vi "Edit Options.vi"(8 "error in (no error)":errorcluster, 11 "Config":T1) -> (0 "error out":errorcluster, 2 "OK?":bool, 3 "Config out":T1)   [LabVIEW 2023, in "VI Properties Editor.lvlib"]
doc: "Displays a window to edit various options present in the tool."
uses:
  VI Properties Editor.lvlib
  CTLs/Config.ctl
panel:
  in  "Abbreviate Names?":bool caption="Abbreviate names"
  in  "Format Bold Tags?":bool caption="Format bold text tags"
  in  "Show Conpane Ctls Only?":bool caption="Show connector pane controls only"
  in  "Confirm Revert All?":bool caption="Confirm Revert All action"
  in  "Confirm Revert?":bool caption="Confirm Revert action"
  in  "Confirm Save All?":bool caption="Confirm Save All action"
  in  "Confirm Save?":bool caption="Confirm Save action"
  in  "Cancel":bool
  in  "OK":bool
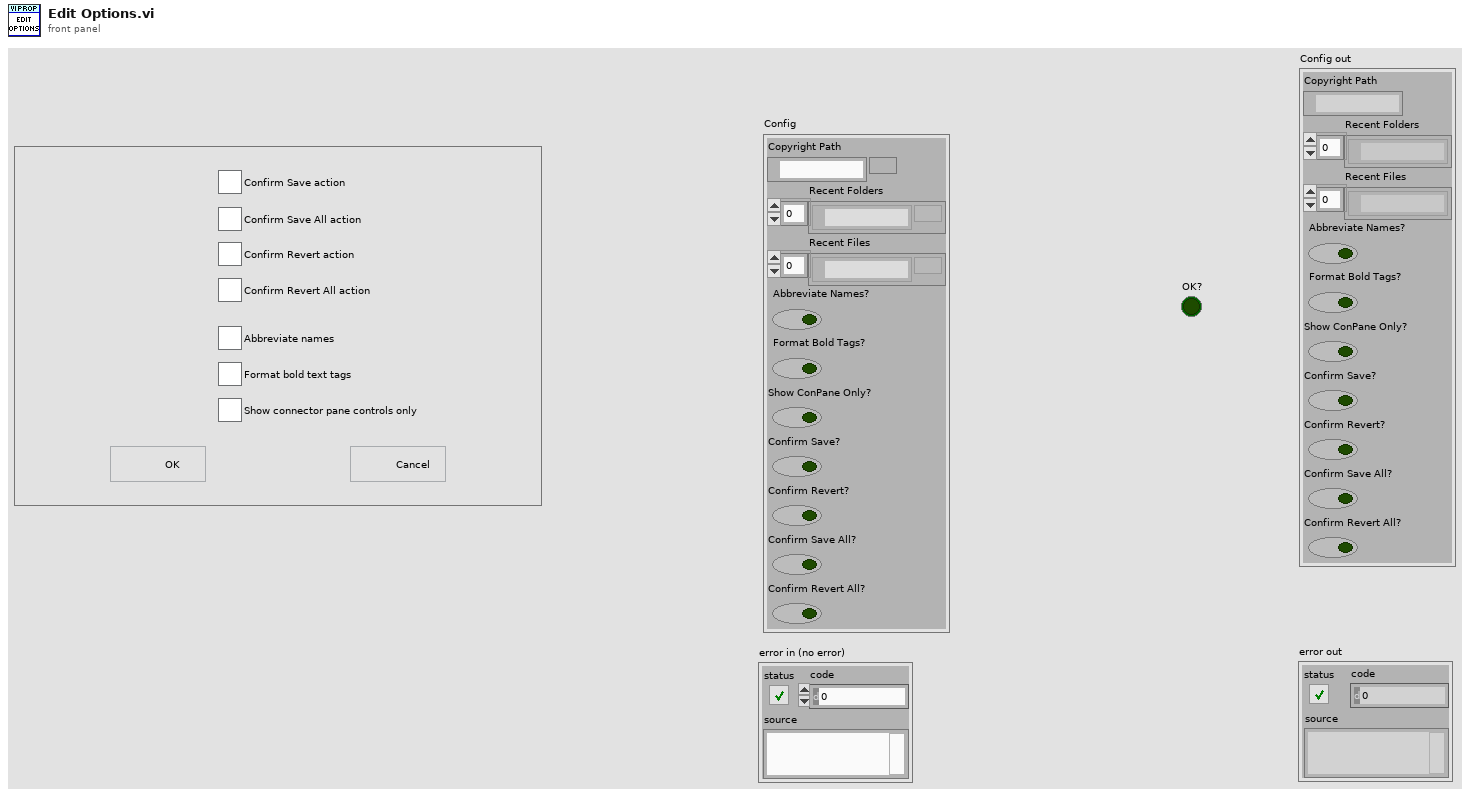
[diagram p1: front panel]
types:
  T1 = typedef "VI Properties Editor.lvlib/Config.ctl" = cluster{"Copyright Path":path, "Recent Folders":path[], "Recent Files":path[], "Abbreviate Names?":bool, "Format Bold Tags?":bool, "Show ConPane Only?":bool, "Confirm Save?":bool, "Confirm Revert?":bool, "Confirm Save All?":bool, "Confirm Revert All?":bool}
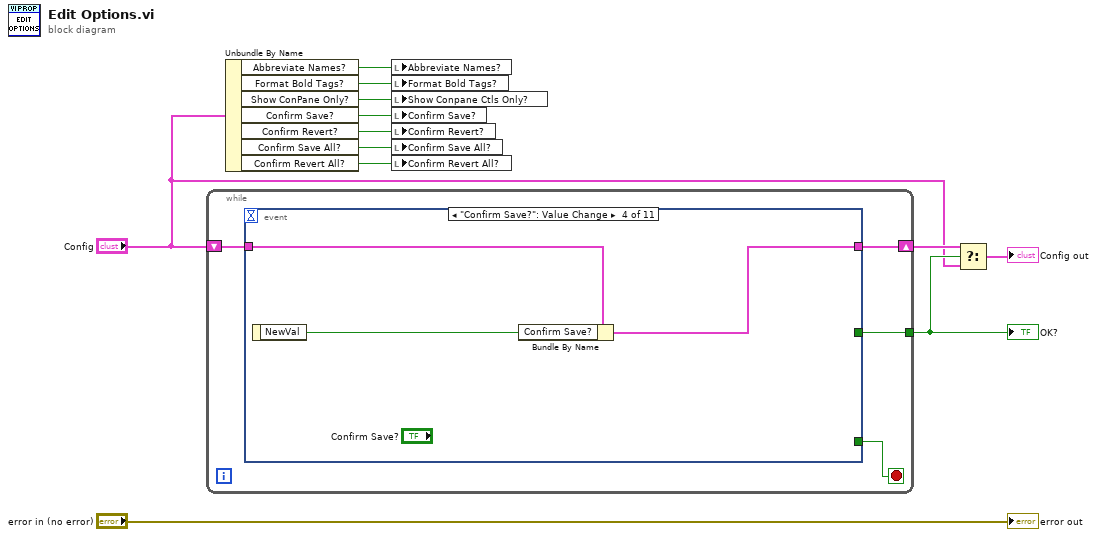
[diagram p0: block diagram]
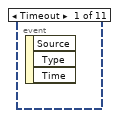
[diagram p2: hidden frame]
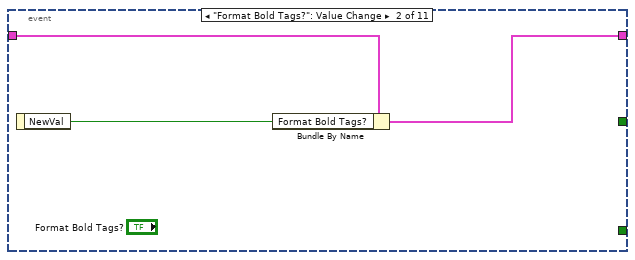
[diagram p3: hidden frame]
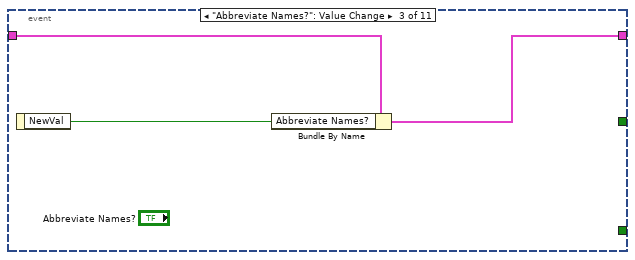
[diagram p4: hidden frame]
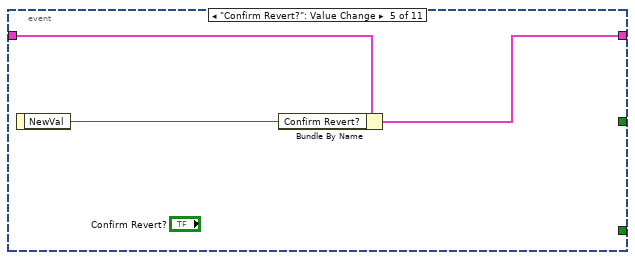
[diagram p5: hidden frame]
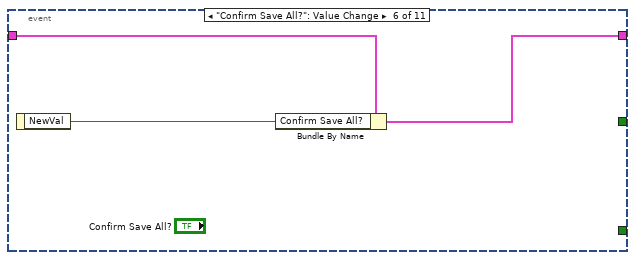
[diagram p6: hidden frame]
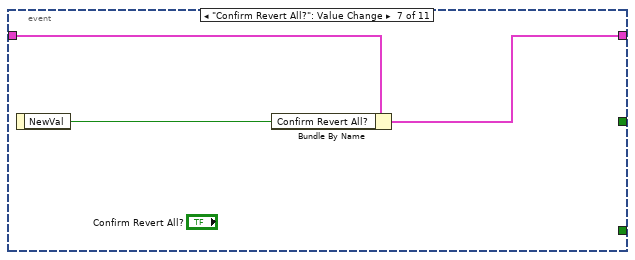
[diagram p7: hidden frame]
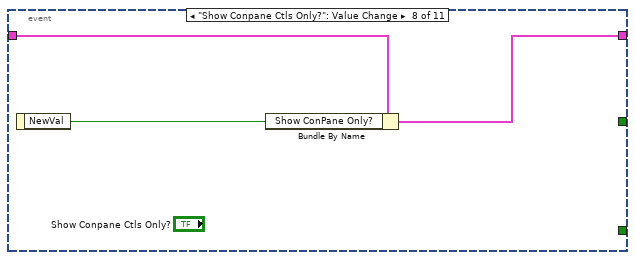
[diagram p8: hidden frame]
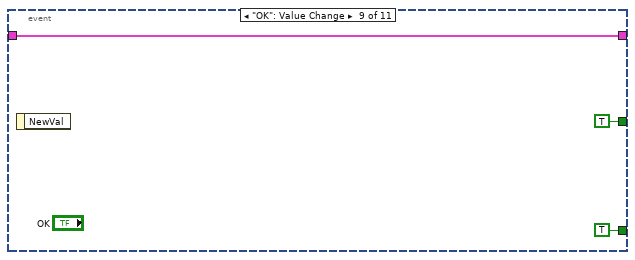
[diagram p9: hidden frame]
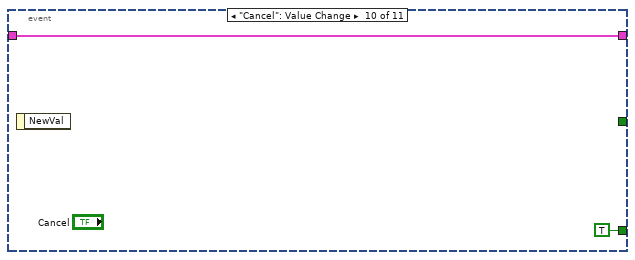
[diagram p10: hidden frame]
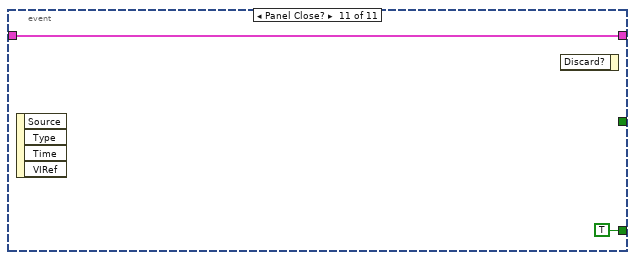
[diagram p11: hidden frame]
diagram:
  n1 = while {
    shift-right: [w15] -> w4
    shift-left: "Config" -> [w16]
    tunnel: [w14] -> w3
    stop <- w13 stop-if-true
    n2 = event shown="[3] \"Confirm Save?\": Value Change" {
      selector: _ -> [_ _ _ _ _ _ _ _ _ _ _]
      dyn-events: _ -> [_ _ _ _ _ _ _ _ _ _ _]
      timeout: _ -> [_ _ _ _ _ _ _ _ _ _ _]
      tunnel: w16 -> [_ w19 w22 w25 w28 w31 w34 w37 w40 w42 w44]
      tunnel: [_ w17 w20 w23 w26 w29 w32 w35 w40 w42 w44] -> w15
      tunnel: [_ _ _ _ _ _ _ _ TRUE ("NewVal") _ _] -> w14
      tunnel: [_ _ _ _ _ _ _ _ TRUE ("NewVal") TRUE ("NewVal") TRUE ("NewVal")] -> w13
      event Timeout {
        n3 = event-data() -> ()  [unwired: 1 in, 3 out]
      }
      event "Format Bold Tags?": Value Change {
        n4 = event-data() -> ("NewVal"=w18:bool)  [unwired: 1 in]
        n5 = Bundle By Name(cluster=w19, "Format Bold Tags?"=w18) -> (w17:T1)
      }
      event "Abbreviate Names?": Value Change {
        n6 = event-data() -> ("NewVal"=w21:bool)  [unwired: 1 in]
        n7 = Bundle By Name(cluster=w22, "Abbreviate Names?"=w21) -> (w20:T1)
      }
      event "Confirm Save?": Value Change {
        n8 = event-data() -> ("NewVal"=w24:bool)  [unwired: 1 in]
        n9 = Bundle By Name(cluster=w25, "Confirm Save?"=w24) -> (w23:T1)
      }
      event "Confirm Revert?": Value Change {
        n10 = event-data() -> ("NewVal"=w27:bool)  [unwired: 1 in]
        n11 = Bundle By Name(cluster=w28, "Confirm Revert?"=w27) -> (w26:T1)
      }
      event "Confirm Save All?": Value Change {
        n12 = event-data() -> ("NewVal"=w30:bool)  [unwired: 1 in]
        n13 = Bundle By Name(cluster=w31, "Confirm Save All?"=w30) -> (w29:T1)
      }
      event "Confirm Revert All?": Value Change {
        n14 = event-data() -> ("NewVal"=w33:bool)  [unwired: 1 in]
        n15 = Bundle By Name(cluster=w34, "Confirm Revert All?"=w33) -> (w32:T1)
      }
      event "Show Conpane Ctls Only?": Value Change {
        n16 = event-data() -> ("NewVal"=w36:bool)  [unwired: 1 in]
        n17 = Bundle By Name(cluster=w37, "Show ConPane Only?"=w36) -> (w35:T1)
      }
      event "OK": Value Change {
        n18 = event-data() -> ()  [unwired: 1 in, 1 out]
      }
      event "Cancel": Value Change {
        n19 = event-data() -> ()  [unwired: 1 in, 1 out]
      }
      event Panel Close? {
        n20 = event-data() -> ()  [unwired: 1 in, 4 out]
        n21 = event-data() -> ()  [unwired: 2 in, 1 out]
      }
    }
  }
  "OK?" <- w3
  n22 = Unbundle By Name("Config") -> ("Abbreviate Names?"=w5:bool, "Format Bold Tags?"=w11:bool, "Show ConPane Only?"=w10:bool, "Confirm Save?"=w9:bool, "Confirm Revert?"=w8:bool, "Confirm Save All?"=w7:bool, "Confirm Revert All?"=w6:bool)
  n23 = local write "Abbreviate Names?"(w5) -> ()
  n24 = local write "Format Bold Tags?"(w11) -> ()
  n25 = local write "Show Conpane Ctls Only?"(w10) -> ()
  n26 = local write "Confirm Save?"(w9) -> ()
  n27 = local write "Confirm Revert?"(w8) -> ()
  n28 = local write "Confirm Save All?"(w7) -> ()
  n29 = local write "Confirm Revert All?"(w6) -> ()
  n30 = Select(t=w4, s=w3, f="Config") -> (s? t:f=→"Config out":T1)
  "error out" <- "error in (no error)"
